vi "Configure Instrument.vi"(8 "error in (no error)":errorcluster, 11 "instrument.PPMS2 in":refnum<class "instrument.PPMS2.lvclass">) -> (0 "error out":errorcluster, 3 "instrument.PPMS2 out":refnum<class "instrument.PPMS2.lvclass">)   [LabVIEW 2016, in "instrument.PPMS2.lvclass"]
uses:
  instrument.PPMS2.lvclass
  <userlib>/LevyLab/Levylab Instruments/Instrument Types/Cryostat/Instrument.Cryostat.lvclass
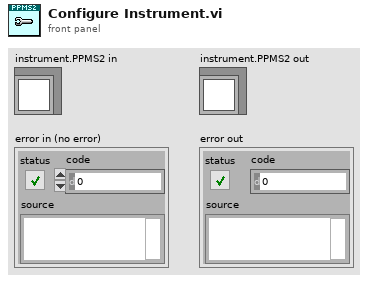
[diagram p1: front panel]
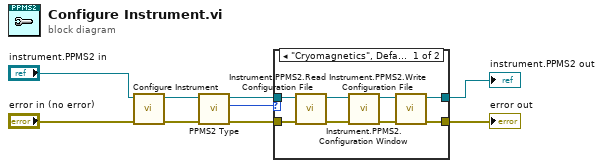
[diagram p0: block diagram]
diagram:
  n1 = call-parent "Configure Instrument.vi"("error in (no error)"="error in (no error)", "Instrument in"="instrument.PPMS2 in") -> ("error out"=w4:errorcluster, "Instrument out"=w3:refnum<class "instrument.PPMS2.lvclass">)  [unwired: 8 in]
  n2 = call "PPMS2 Type.vi"("error in (no error)"=w4, "instrument.PPMS2 in"=w3) -> ("error out"=w1:errorcluster, "PPMS \"Type\""=w5:enum16{"Cryomagnetics", "QD only"}, "instrument.PPMS2 out"=w2:refnum<class "instrument.PPMS2.lvclass">)  [unwired: 7 in]
  n3 = case shown="\"Cryomagnetics\", Default" w5 {
    tunnel: w1 -> [w17 w18]
    tunnel: w2 -> [w16 w19]
    tunnel: [w11 w18] -> w7
    tunnel: [w10 w19] -> w6
    frame "Cryomagnetics", Default {
      n4 = call-dynamic "Instrument.PPMS2.Read Configuration File.vi"("error in (no error)"=w17, "instrument.PPMS2 in"=w16) -> ("error out"=w14:errorcluster, "instrument.PPMS2 out"=w15:refnum<class "instrument.PPMS2.lvclass">)  [unwired: 8 in]
      n5 = call-dynamic "Instrument.PPMS2.Configuration Window.vi"("error in (no error)"=w14, "instrument.PPMS2 in"=w15) -> ("error out"=w12:errorcluster, "instrument.PPMS2 out"=w13:refnum<class "instrument.PPMS2.lvclass">)  [unwired: 8 in]
      n6 = call-dynamic "Instrument.PPMS2.Write Configuration File.vi"("error in (no error)"=w12, "instrument.PPMS2 in"=w13) -> ("error out"=w11:errorcluster, "instrument.PPMS2 out"=w10:refnum<class "instrument.PPMS2.lvclass">)  [unwired: 8 in]
    }
    frame "QD only" {
    }
  }
  "error out" <- w7
  "instrument.PPMS2 out" <- w6
